vi "Pre Launch Init.vi"(11 "Event Source In":refnum<class "Event Source Actor.lvclass">) -> (0 "Error Out":errorcluster, 3 "Event Source Out":refnum<class "Event Source Actor.lvclass">)   [LabVIEW 2021, in "EventSourceActor.lvlib" / "Event Source.lvlib" / "Event Source Actor.lvclass"]
doc: "(<B>Filename</B>: Actor Framework.lvlib:Actor.lvclass:Pre Launch Init.vi)\n\nDefines behavior that occurs after the Launch Nested Actor method is invoked but before the actor's Actor Core method begins running.\n\nBy default, this method does nothing. A descendant class may override it to define behavior."
uses:
  Event Source Actor.lvclass
  <vilib>/ActorFramework/Message Enqueuer/Message Enqueuer.lvclass
  Event Source Actor.lvclass/Event Source Actor.ctl
  <vilib>/ActorFramework/Actor/Actor.lvclass
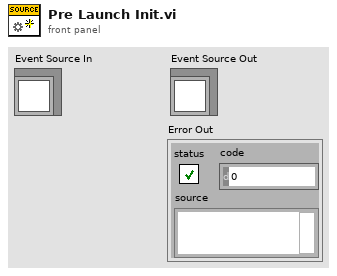
[diagram p1: front panel]
types:
  T1 = map{string, set{refnum<class "Message Enqueuer.lvclass">}}
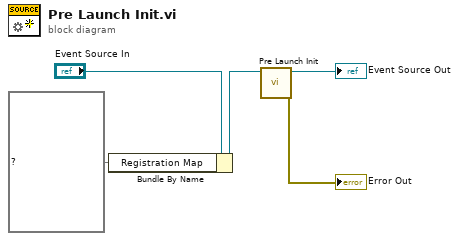
[diagram p0: block diagram]
diagram:
  n1 = Bundle By Name(cluster="Event Source In", "Registration Map"=T1 {}) -> (w3:refnum<class "Event Source Actor.lvclass">)
  n2 = call-parent "Pre Launch Init.vi"("Actor in"=w3) -> ("error out"=→"Error Out":errorcluster, "Actor out"=→"Event Source Out":refnum<class "Event Source Actor.lvclass">)  [unwired: 9 in]
